vi "DELETE (SubVI).vi"(8 "error in (no error)":errorcluster, 9 "input 1":string, 10 "Boolean":bool, 11 "Refnum in":T1) -> (0 "error out":errorcluster, 3 "Refnum out":T1)   [LabVIEW 2024]
uses:
  <vilib>/addons/database/Connection.llb/Conn ObjectReference.ctl
  <vilib>/addons/database/Connection.llb/Conn Execute.vi
  <vilib>/addons/database/NI_Database_API.lvlib
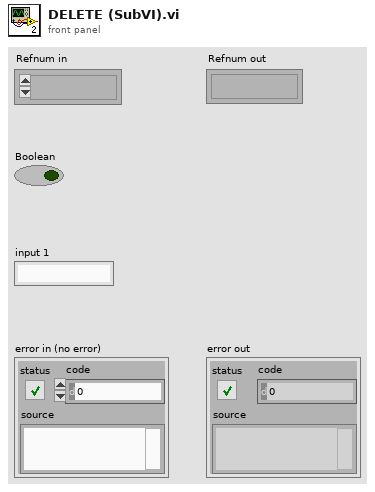
[diagram p1: front panel]
types:
  T1 = typedef "NI_Database_API.lvlib/Conn ObjectReference.ctl" = refnum<k1>
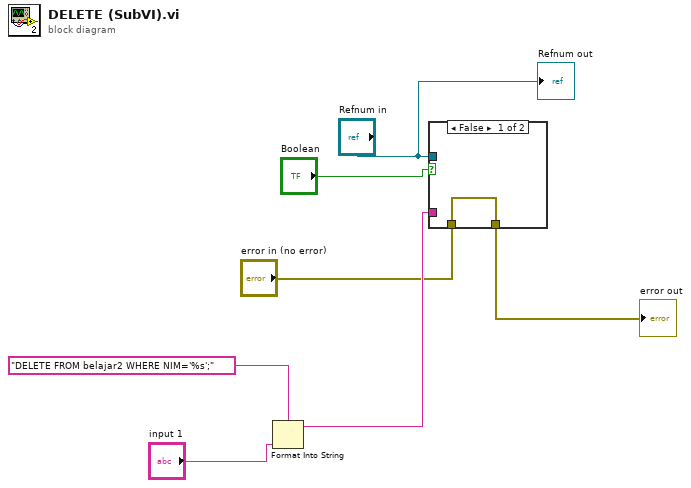
[diagram p0: block diagram]
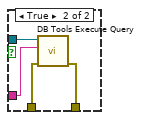
[diagram p2: hidden frame]
diagram:
  n1 = Format Into String(format string="DELETE FROM belajar2 WHERE NIM='%s';", "input 1") -> (resulting string=w7:string)  [unwired: 2 in, 1 out]
  n2 = case shown="False" "Boolean" {
    tunnel: "Refnum in" -> [_ w12]
    tunnel: "error in (no error)" -> [w8 w11]
    tunnel: [w8 w10] -> w3
    tunnel: w7 -> [_ w9]
    frame False {
    }
    frame True {
      n3 = call-poly <vilib>:"DB Tools Execute Query.vi"("error in (no error)"=w11, "SQL query"=w9, "connection reference"=w12) -> ("error out"=w10:errorcluster)  [unwired: 5 in, 1 out]
    }
  }
  "error out" <- w3
  "Refnum out" <- "Refnum in"
